vi "Output State (Set).vi"(6 "ISOBUS address":T3=-1 caption="ISOBUS address (-1)", 8 "error in":errorcluster, 9 "Output to Set":u8, 10 "State":string, 11 "Mercury Reference In":T4) -> (0 "error out":errorcluster, 2 "Response":T1, 3 "Mercury Reference Out":T4, 4 "Valid?":T2)   [LabVIEW 2016, in "Mercury iXX.lvlib" / "Auxiliary.lvlib"]
doc: "Set the output state of an output."
uses:
  Auxiliary.lvlib
  Controls/Mercury Reference.ctl
  Controls/Comms Transport Layer.ctl
  Private/Controls/Query Dynamic Reference.ctl
  Controls/ISOBus Address.ctl
  Controls/Is Valid LED.ctl
  Controls/Response String.ctl
  Private/Controls/Command Verbs.ctl
  Mercury iXX.lvlib
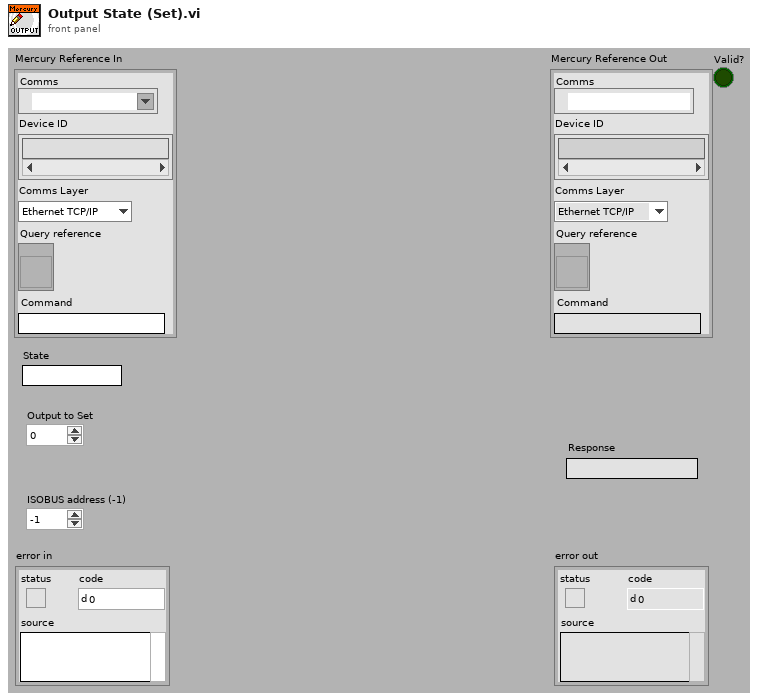
[diagram p1: front panel]
types:
  T1 = typedef "Mercury iXX.lvlib/Response String.ctl" = string
  T2 = typedef "Mercury iXX.lvlib/Is Valid LED.ctl" = bool
  T3 = typedef "Mercury iXX.lvlib/ISOBus Address.ctl" = i32
  T4 = typedef "Mercury iXX.lvlib/Mercury Reference.ctl" = cluster{"Comms":refnum<visa-resource-name>, "Device ID":string[], "Comms Layer":T5, "Command":string, "Query reference":T6}
  T5 = typedef "Mercury iXX.lvlib/Comms Transport Layer.ctl" = enum16{"Ethernet TCP/IP", "USB", "ISOBus - RS-232", "GPIB"}
  T6 = typedef "Mercury iXX.lvlib/Query Dynamic Reference.ctl" = refnum<vi>
  T7 = typedef "Mercury iXX.lvlib/Command Verbs.ctl" = string
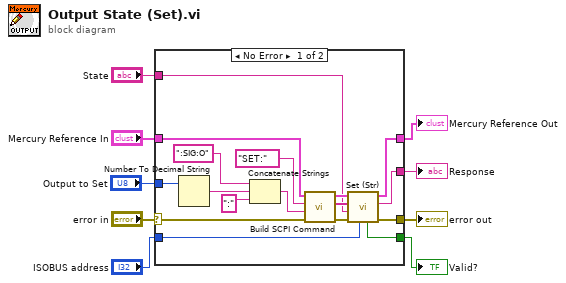
[diagram p0: block diagram]
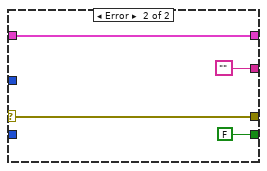
[diagram p2: hidden frame]
diagram:
  n1 = case shown="No Error" "error in" {
    selector: "error in" -> [w15 w29]
    tunnel: "ISOBUS address" -> [w26 _]
    tunnel: [w25 T2 FALSE ("Valid?")] -> w4
    tunnel: [w24 w30] -> w6
    tunnel: [w23 w29] -> w3
    tunnel: [w22 ""] -> w5
    tunnel: "Mercury Reference In" -> [w19 w30]
    tunnel: "State" -> [w14 _]
    tunnel: "Output to Set" -> [w12 _]
    frame No Error {
      n2 = Number To Decimal String(number=w12) -> (decimal integer string=w11:string)  [unwired: 1 out]
      n3 = Concatenate Strings(":SIG:O" ("Command"), w11, ":" ("string")) -> (w13:string)
      n4 = call "Build SCPI Command.vi"("error in"=w15, "Noun(s)"=w13, "Verb"=T7 "SET:", "Mercury Reference In"=w19) -> ("error out"=w17:errorcluster, "SCPI Message(s)"=w16:string[], "Mercury Reference Out"=w18:T4)  [unwired: 5 out]
      n5 = call "Set (Str).vi"("ISOBUS address"=w26, "error in"=w17, "Command Value (Str)"=w14, "SCPI Message(s)"=w16, "Mercury Reference In"=w18) -> ("error out"=w23:errorcluster, "Response"=w22:T1, "Mercury Reference Out"=w24:T4, "Valid?"=w25:T2)  [unwired: 1 in, 2 out]
    }
    frame Error {
    }
  }
  "Mercury Reference Out" <- w6
  "Valid?" <- w4
  "error out" <- w3
  "Response" <- w5
